vi "Compact if necessary.vi"(1 "bytestream":refnum<class "Bytestream.lvclass">) -> (0 "bytestream out":refnum<class "Bytestream.lvclass">)   [LabVIEW 2020, in "NI_Bytestream.lvlib" / "Bytestream.lvclass"]
uses:
  <vilib>/Array/Bytestream/Bytestream.lvclass
  <vilib>/Array/Bytestream/Bytestream.lvclass/Bytestream.ctl
  <vilib>/Array/Bytestream/Count Datums.vi
  <vilib>/Array/Bytestream/Get Logical Datum.vi
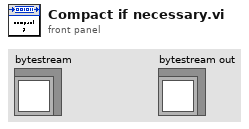
[diagram p1: front panel]
types:
  T1 = typedef "NI_Bytestream.lvlib/Bytestream.lvclass/Datum.ctl" = cluster{"array":u8[], "index":i32}
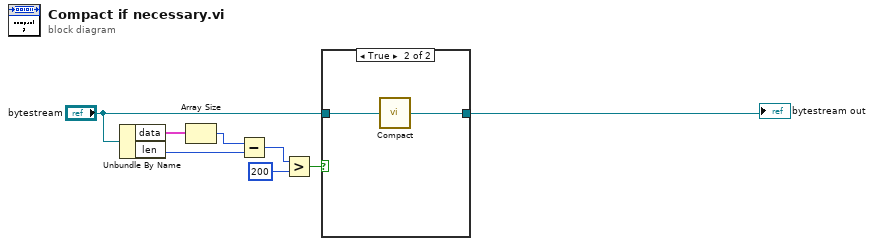
[diagram p0: block diagram]
diagram:
  n1 = Unbundle By Name("bytestream") -> ("data"=w8:T1[], "len"=w6:i32)
  n2 = Array Size(array=w8) -> (size(s)=w7:i32)
  n3 = Subtract(x=w7, y=w6) -> (x-y=w5:i32)
  n4 = Greater?(x=w5, y=200) -> (0:w3:bool)
  n5 = case shown="True" w3 {
    tunnel: "bytestream" -> [w9 w11]
    tunnel: [w9 w10] -> w1
    frame False {
    }
    frame True {
      n6 = call <vilib>:"Compact.vi"("bytestream"=w11) -> ("bytestream out"=w10:refnum<class "Bytestream.lvclass">)
    }
  }
  "bytestream out" <- w1
